vi "cw_1_1.vi"() -> ()   [LabVIEW 2022 SP3]
panel:
  out "String 1":string
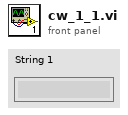
[diagram p1: front panel]
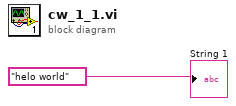
[diagram p0: block diagram]
diagram:
  "String 1" <- "helo world"
